vi "autostage-coordinates-minmax.vi"(0 "coordinates":dbl[][](array[numeric])) -> (1 "x-max":u16, 2 "x-min":u16, 3 "y-max":u16, 4 "y-min":u16)   [LabVIEW 2015]
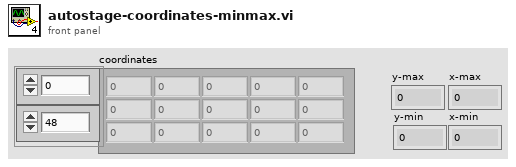
[diagram p1: front panel]
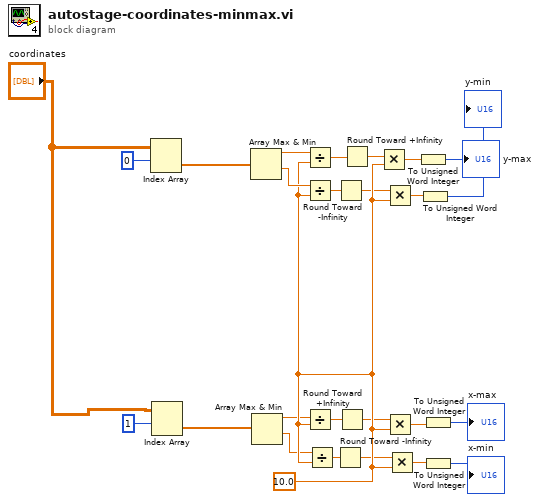
[diagram p0: block diagram]
diagram:
  w17 = 10.0 ("y")
  n1 = Index Array(array="coordinates", index (row)=0) -> (element=w23:dbl[])  [unwired: 1 in]
  n2 = Index Array(array="coordinates", index (row)=1) -> (element=w22:dbl[])  [unwired: 1 in]
  n3 = Array Max & Min(array=w23) -> (max value=w21:dbl, min value=w18:dbl)  [unwired: 2 out]
  n4 = Array Max & Min(array=w22) -> (max value=w14:dbl, min value=w9:dbl)  [unwired: 2 out]
  n5 = Divide(x=w21, y=w17) -> (x/y=w19:dbl)
  n6 = Divide(x=w18, y=w17) -> (x/y=w16:dbl)
  n7 = Divide(x=w14, y=w17) -> (x/y=w13:dbl)
  n8 = Divide(x=w9, y=w17) -> (x/y=w12:dbl)
  n9 = Round Toward -Infinity(1:w12) -> (0:w10:dbl)
  n10 = Round Toward -Infinity(1:w16) -> (0:w15:dbl)
  n11 = Round Toward +Infinity(x=w13) -> (ceil(x): smallest int >= x=w11:dbl)
  n12 = Round Toward +Infinity(x=w19) -> (ceil(x): smallest int >= x=w20:dbl)
  n13 = Multiply(x=w20, y=w17) -> (x*y=w8:dbl)
  n14 = Multiply(x=w15, y=w17) -> (x*y=w7:dbl)
  n15 = Multiply(x=w11, y=w17) -> (x*y=w6:dbl)
  n16 = Multiply(x=w10, y=w17) -> (x*y=w5:dbl)
  n17 = To Unsigned Word Integer(number=w8) -> (unsigned 16bit integer=→"y-max":u16)
  n18 = To Unsigned Word Integer(number=w7) -> (unsigned 16bit integer=→"y-min":u16)
  n19 = To Unsigned Word Integer(number=w6) -> (unsigned 16bit integer=→"x-max":u16)
  n20 = To Unsigned Word Integer(number=w5) -> (unsigned 16bit integer=→"x-min":u16)
